vi "Lorentzian model function.vi"(3 "output control":T1, 4 "data":variant, 5 "X":dbl[](array[numeric]), 6 "a":dbl[](array[numeric])) -> (0 "error out":errorcluster, 1 "f'(X,a)":dbl[][](array[numeric]), 2 "f(X,a)":dbl[](array[numeric]))   [LabVIEW 2014]
doc: "This template is the starting point for creating a model function to be passed to the Nonlinear Curve Fit.vi."
uses:
  <vilib>/gmath/NumericalOptimization/LM_output select.ctl
  <vilib>/gmath/NI_Gmath.lvlib
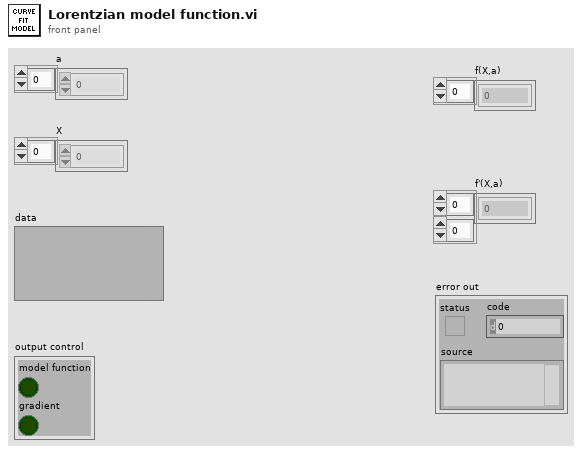
[diagram p1: front panel]
types:
  T1 = typedef "NI_Gmath.lvlib/LM_output select.ctl" = cluster{"model function":bool, "gradient":bool}
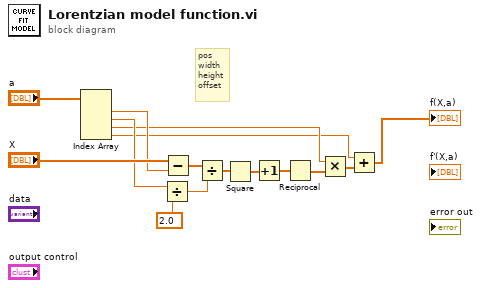
[diagram p0: block diagram]
diagram:
  # "pos\nwidth\nheight\noffset"
  n1 = Index Array(array="a") -> (element #1=w8:dbl, element #2=w7:dbl, element #3=w4:dbl, element #4=w2:dbl)  [unwired: 4 in]
  n2 = Divide(x=w7, y=2.0) -> (x/y=w6:dbl)
  n3 = Subtract(x="X", y=w8) -> (x-y=w11:dbl[])
  n4 = Divide(x=w11, y=w6) -> (x/y=w14:dbl[])
  n5 = Square(x=w14) -> (x^2=w13:dbl[])
  n6 = Increment(x=w13) -> (x+1=w12:dbl[])
  n7 = Reciprocal(x=w12) -> (1/x=w5:dbl[])
  n8 = Multiply(x=w4, y=w5) -> (x*y=w3:dbl[])
  n9 = Add(x=w2, y=w3) -> (x+y=→"f(X,a)":dbl[])
